vi "Stop Core.vi"(10 "final error code":i32, 11 "TestBench in":refnum<class "TestBench.lvclass">) -> (3 "TestBench out":refnum<class "TestBench.lvclass">)   [LabVIEW 2019, in "TestBench.lvlib" / "TestBench.lvclass"]
uses:
  TestBench.lvclass
  <vilib>/ActorFramework/Actor/Actor.lvclass
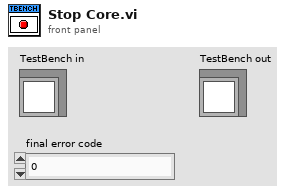
[diagram p1: front panel]
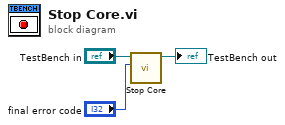
[diagram p0: block diagram]
diagram:
  n1 = call-parent "Stop Core.vi"("final error code"="final error code", "Actor in"="TestBench in") -> ("Actor out"=→"TestBench out":refnum<class "TestBench.lvclass">)  [unwired: 9 in]
